vi "SVM_통합버전.vi"(8 "svm_parameter":T1={"svm_type"=0, "kernel_type"=3, "degree"=3, "gamma"=0.07, "coef0"=0.0, "cache_size"=100.0, "epsilon"=0.001, "C"=1.0, "nr_weight"=0, "weight_label"=[1, 12], "Weight (C(class i))"=[1.0, 1.0], "nu"=0.5, "p"=0.1, "Shrinking"=1, "probability"=1} {"p" format="%.4f"; "nu" format="%.4f"; "Weight (C(class i))" format="%.2f"; "C" format="%.2f"; "epsilon" format="%.4f"; "cache_size" format="%.2f"; "coef0" format="%.2f"; "gamma" format="%.5f"; "kernel_type" items=["Linear", "Poly", "RBF", "Sigmoid"]; "svm_type" items=["C-SVC", "Nu-SVC", "One-class SVM", "epsilon-SVR", "nu-SVR"]}, 9 "ModelFileName":string="C:\\\\WORK\\\\RBFModel", 10 "ERP_Parameters_of_Target":dbl[][](array[numeric]) format="%0.3f", 11 "ERP_Parameters_of_Nontarget":dbl[][](array[numeric]) format="%0.3f") -> ()   [LabVIEW 2013]
panel:
  out "Length":i32=12
  # "Results"
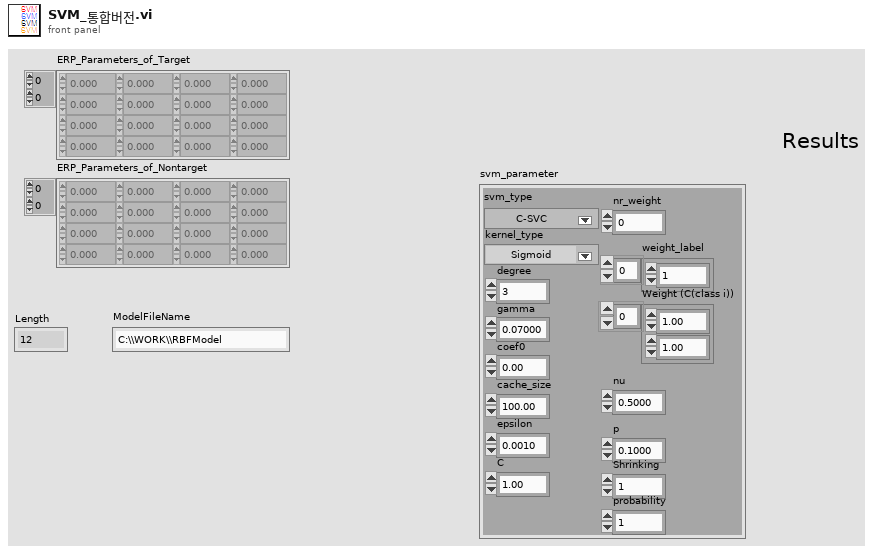
[diagram p1: front panel]
types:
  T1 = cluster{"svm_type":i16, "kernel_type":i16, "degree":i16, "gamma":dbl, "coef0":dbl, "cache_size":dbl, "epsilon":dbl, "C":dbl, "nr_weight":i16, "weight_label":i16[], "Weight (C(class i))":dbl[], "nu":dbl, "p":dbl, "Shrinking":i16, "probability":i16}
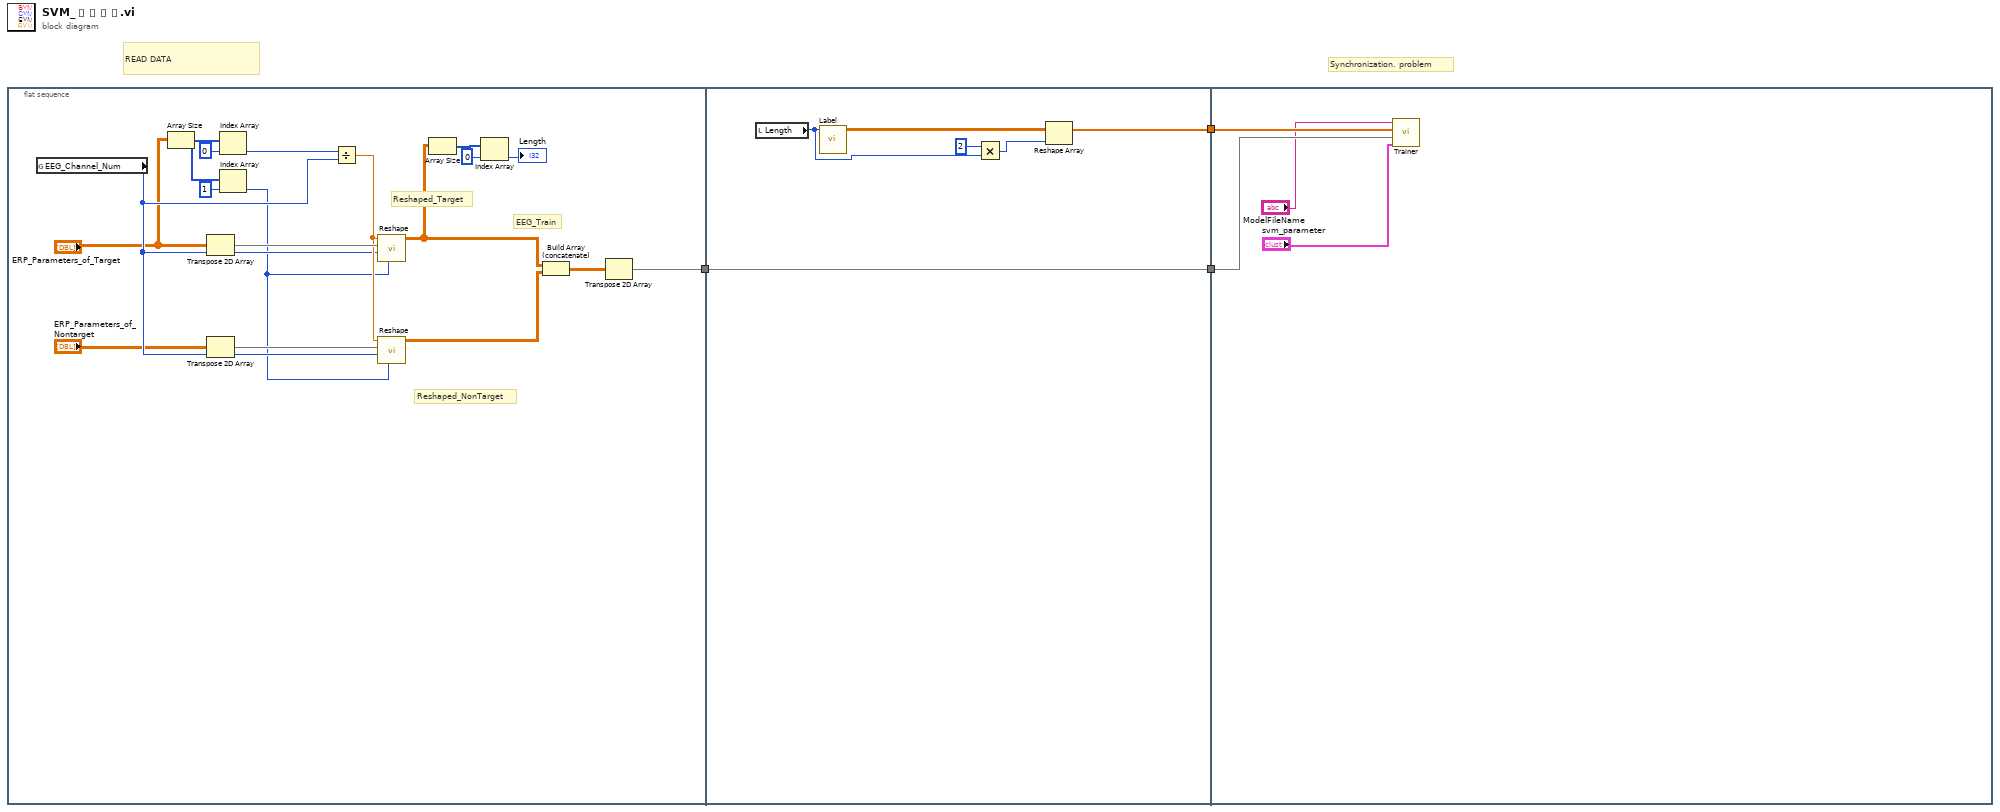
[diagram p0: block diagram]
diagram:
  # "Synchronization. problem"
  # "READ DATA"
  n1 = flat-sequence {
    tunnel: [w12] -> w3
    tunnel: w3 -> [w22]
    tunnel: [w22] -> w2
    tunnel: [w26] -> w1
    tunnel: w2 -> [w30]
    tunnel: w1 -> [w31]
    frame #0 {
      # "EEG_Train"
      # "Reshaped_NonTarget"
      # "Reshaped_Target"
      n2 = global read "Control_Panel.vi" "EEG_Channel_Num"() -> (w10:i32)
      n3 = Array Size(array="ERP_Parameters_of_Target") -> (size(s)=w19:i32[])
      n4 = Transpose 2D Array(2D array="ERP_Parameters_of_Target") -> (transposed array=w15:dbl[][])
      n5 = Transpose 2D Array(2D array="ERP_Parameters_of_Nontarget") -> (transposed array=w14:dbl[][])
      n6 = Index Array(array=w19, index=0) -> (element=w18:i32)
      n7 = Index Array(array=w19, index=1) -> (element=w9:i32)
      n8 = Divide(x=w18, y=w10) -> (x/y=w11:dbl)
      n9 = call "Reshape.vi"("Numeric"=w9, "EEG_Channel_Num"=w10, "all rows"=w15, "Numeric 2"=w11) -> ("Array"=w8:dbl[][])  [unwired: 7 in]
      n10 = call "Reshape.vi"("Numeric"=w9, "EEG_Channel_Num"=w10, "all rows"=w14, "Numeric 2"=w11) -> ("Array"=w7:dbl[][])  [unwired: 7 in]
      n11 = Array Size(array=w8) -> (size(s)=w16:i32[])
      n12 = Index Array(array=w16, index=0) -> (element=→"Length":i32)
      n13 = Build Array (concatenate)(w8, w7) -> (w6:dbl[][])
      n14 = Transpose 2D Array(2D array=w6) -> (transposed array=w12:dbl[][])
    }
    frame #1 {
      n15 = local read "Length"() -> (w24:i32)
      n16 = call "Label.vi"("Numeric"=w24) -> ("Array"=w27:dbl[][])  [unwired: 10 in]
      n17 = Multiply(x=2, y=w24) -> (x*y=w25:i32)
      n18 = Reshape Array(w27, w25) -> (w26:dbl[])
    }
    frame #2 {
      n19 = call "Trainer.vi"("svm_parameter"="svm_parameter", "attributes"=w30, "Lables"=w31, "ModelFileName"="ModelFileName") -> ()
    }
  }
